vi "Add Meas Plugin Indicators - Single Converter.vi"(11 "error in":errorcluster) -> (15 "error out":errorcluster)   [LabVIEW 2021, in "Converter.lvlib"]
uses:
  Converter.lvlib
  Converter Reusables/Converter Reusables.lvlib
  Path Functions/Path Functions.lvlib
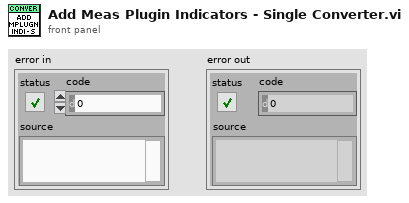
[diagram p1: front panel]
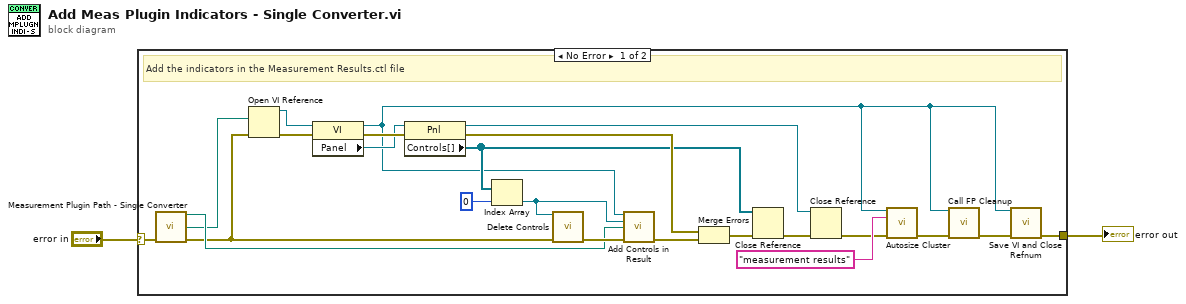
[diagram p0: block diagram]
diagram:
  n1 = case shown="No Error" "error in" {
    selector: "error in" -> [w5 w26]
    tunnel: [w3 w26] -> w2
    frame No Error {
      # "Add the indicators in the Measurement Results.ctl file"
      n2 = call "Measurement Plugin Path - Single Converter.vi"("error in"=w5) -> ("new code module"=w7:path, "result control"=w6:path, "error out"=w4:errorcluster)  [unwired: 2 in, 10 out]
      n3 = Open VI Reference(vi path=w6, error in (no error)=w4) -> (vi reference=w11:refnum<vi>, error out=w21:errorcluster)  [unwired: 4 in]
      n4 = property class="VI"(reference=w11, error in=w21) -> (reference out=w10:refnum<vi>, error out=w25:errorcluster, "Panel"=w22:refnum<vi>)
      n5 = property class="Pnl"(reference=w22, error in=w25) -> (reference out=w16:refnum<vi>, error out=w15:errorcluster, "Controls[]"=w14:refnum<vi>[])
      n6 = Index Array(array=w14, index=0) -> (element=w9:refnum<vi>)
      n7 = call "Delete Controls.vi"("control in"=w9, "error in"=w4) -> ("error out"=w8:errorcluster)  [unwired: 13 in]
      n8 = call "Add Controls in Result.vi"("vi reference"=w10, "result cluster"=w9, "new code module"=w7, "error in"=w8) -> ("error out"=w23:errorcluster)  [unwired: 11 in]
      n9 = Merge Errors(w15, w23) -> (w13:errorcluster)
      n10 = Close Reference(reference=w14, error in (no error)=w13) -> (error out=w12:errorcluster)
      n11 = Close Reference(reference=w16, error in (no error)=w12) -> (error out=w19:errorcluster)
      n12 = call "Autosize Cluster.vi"("vi refnum"=w10, "name"="measurement results" ("name/order"), "error in"=w19) -> ("error out"=w18:errorcluster)  [unwired: 12 in]
      n13 = call "Call FP Cleanup.vi"("vi"=w10, "error in"=w18) -> ("error out"=w17:errorcluster)  [unwired: 13 in]
      n14 = call "Save VI and Close Refnum.vi"("vi refnum"=w10, "error in"=w17) -> ("error out"=w3:errorcluster)  [unwired: 13 in]
    }
    frame Error {
    }
  }
  "error out" <- w2
